vi "Build Param Properties.vi"(0 "Parameter":T3, 2 "HardwareChannel":i32, 4 "Word":bool[](array[boolean]), 5 "error in (no error)":errorcluster) -> (7 "signed":bool, 8 "Prop Names":string[](array[string]), 9 "numberBits":i32, 10 "Prop Values":variant[](array[variant]), 11 "startBit":i32, 13 "scaleFactor":dbl, 14 "Channel":T1, 16 "name":string, 18 "error out":errorcluster, 19 "scaleOffset":dbl)   [LabVIEW 2017, in "Ballard Arinc-429 System Explorer.lvlib"]
uses:
  Ballard Arinc-429 System Explorer.lvlib
  Parse Parameters File/XML_Parameter.ctl
  <vilib>/NI Veristand/Custom Device API/Custom Device Channel.ctl
  <vilib>/NI Veristand/Custom Device API/Custom Device Channel Type.ctl
  Shared/Controls and Global/Global.vi
  Shared/Ballard Arinc-429 Shared.lvlib
  <vilib>/NI Veristand/Custom Device API/Custom Device API.lvlib
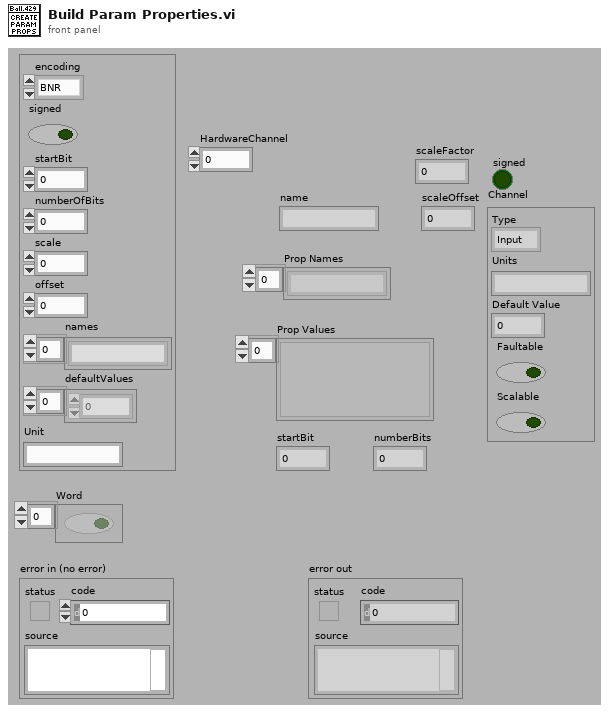
[diagram p1: front panel]
types:
  T1 = typedef "Custom Device API.lvlib/Custom Device Channel.ctl" = cluster{"Type":T2, "Units":string, "Default Value":dbl, "Faultable":bool, "Scalable":bool}
  T2 = typedef "Custom Device API.lvlib/Custom Device Channel Type.ctl" = enum16{"Input", "Output"}
  T3 = typedef "XML_Parameter.ctl" = cluster{"encoding":enum16{"BNR", "BCD", "Discrete"}, "signed":bool, "startBit":i32, "numberOfBits":i32, "scale":dbl, "offset":dbl, "names":string[], "defaultValues":dbl[], "Unit":string}
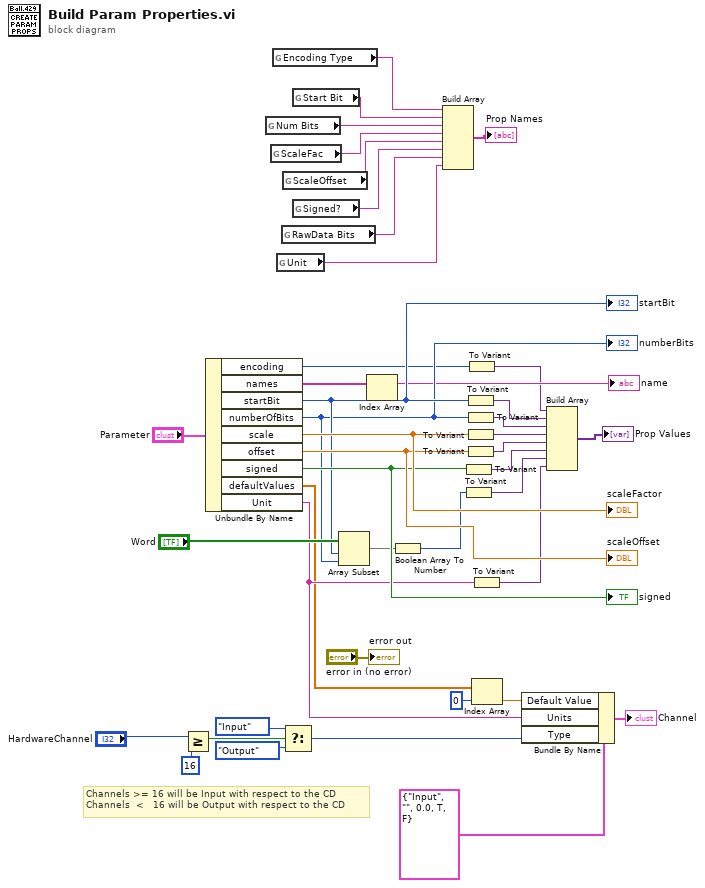
[diagram p0: block diagram]
diagram:
  # "Channels >= 16 will be Input with respect to the CD\nChannels  <   16 will be Output with respect to the CD"
  n1 = Greater Or Equal?(x="HardwareChannel", y=16) -> (x >= y?=w14:bool)
  n2 = Unbundle By Name("Parameter") -> ("encoding"=w7:enum16{"BNR", "BCD", "Discrete"}, "names"=w42:string[], "startBit"=w22:i32, "numberOfBits"=w21:i32, "scale"=w33:dbl, "offset"=w32:dbl, "signed"=w28:bool, "defaultValues"=w2:dbl[], "Unit"=w5:string)
  "startBit" <- w22
  "numberBits" <- w21
  "scaleOffset" <- w32
  "scaleFactor" <- w33
  "signed" <- w28
  n3 = global read "Global.vi" "Num Bits"() -> (w38:string)
  n4 = global read "Global.vi" "ScaleFac"() -> (w36:string)
  n5 = global read "Global.vi" "Encoding Type"() -> (w8:string)
  n6 = global read "Global.vi" "Unit"() -> (w10:string)
  n7 = global read "Global.vi" "RawData Bits"() -> (w25:string)
  n8 = global read "Global.vi" "ScaleOffset"() -> (w30:string)
  n9 = Select(t=Custom_Device_Channel_Type."Input" ("Type"), s=w14, f=Custom_Device_Channel_Type."Output" ("Type")) -> (s? t:f=w11:T2)
  n10 = global read "Global.vi" "Start Bit"() -> (w37:string)
  n11 = global read "Global.vi" "Signed?"() -> (w29:string)
  n12 = Array Subset(array="Word", index=w22, length=w21) -> (w20:bool[])
  n13 = Index Array(array=w42) -> (element=→"name":string)  [unwired: 1 in]
  n14 = Boolean Array To Number(Boolean array=w20) -> (number=w19:u32)
  n15 = Build Array(w8, w37, w38, w36, w30, w29, w25, w10) -> (→"Prop Names":string[])
  n16 = To Variant(anything=w28) -> (Variant=w27:variant)
  n17 = To Variant(anything=w19) -> (Variant=w24:variant)
  n18 = To Variant(anything=w22) -> (Variant=w41:variant)
  n19 = To Variant(anything=w21) -> (Variant=w40:variant)
  n20 = To Variant(anything=w33) -> (Variant=w35:variant)
  n21 = To Variant(anything=w32) -> (Variant=w31:variant)
  n22 = To Variant(anything=w7) -> (Variant=w6:variant)
  n23 = To Variant(anything=w5) -> (Variant=w4:variant)
  n24 = Index Array(array=w2, index=0) -> (element=w3:dbl)
  n25 = Bundle By Name(cluster=T1 {"Type"=enum."Input", "Units"="", "Default Value"=0.0, "Faultable"=TRUE, "Scalable"=FALSE} ("Channel"), "Default Value"=w3, "Units"=w5, "Type"=w11) -> (→"Channel":T1)
  n26 = Build Array(w6, w41, w40, w35, w31, w27, w24, w4) -> (→"Prop Values":variant[])
  "error out" <- "error in (no error)"
